vi "Drive Controller.vi"(8 "error in":errorcluster) -> ()   [LabVIEW 2020]
doc: "This VI executes continuously carrying out the current operation and responding to updates or new operation requests. It will often contain the timing or control code that is difficult to place directly in TeleOp. This VI generally opens all sensors and motors and isolates the rest of the robot code from knowing implementation details of how the operations are carried out."
uses:
  <vilib>/Rock Robotics/WPI/Framework/Completion Status.ctl
  Drive Setpoints.ctl
  Drive Operations.ctl
  Dawgma Programming Library/Controls/PurePursuit/RobotNeededPathData.ctl
  <vilib>/Rock Robotics/WPI/ThirdParty/REV Robotics/REVLib/Typedef/Spark MAX Sensor Type.ctl
  <vilib>/Rock Robotics/WPI/ThirdParty/REV Robotics/REVLib/Typedef/Spark MAX Idle Mode.ctl
  <vilib>/Rock Robotics/WPI/DriverStation/WPI_DriverStationRobotMode2.ctl
  <vilib>/Rock Robotics/WPI/ThirdParty/Sensors/navX/_TypeDefs/FRIC_navX_DeviceNumbersTypeDef.ctl
  <vilib>/Rock Robotics/WPI/ThirdParty/REV Robotics/REVLib/Typedef/Spark MAX Control Type.ctl
  Dawgma Programming Library/Controls/PurePursuit/PathFileData.ctl
  <vilib>/Rock Robotics/Network Tables/NT Write Variant.vi
  Configuration/Constants.vi
  <vilib>/Rock Robotics/Network Tables/NT Read Number.vi
  <vilib>/Rock Robotics/WPI/ThirdParty/Sensors/navX/_Processing Loop/FRIC_navX_Internal_SPI_ProcessingLoop.vi
panel:
  in  "Vel Convert":dbl=0.01786
  in  "Zero Encoders":bool
  out "Actual Angle":dbl=-174.33
  in  "Reset Loc & Ang":bool
  in  "Drive Conversion":dbl=1.75
  in  "SensorData":T1
  out "Graph":cluster{cluster{"x":dbl, "y":dbl}[]}[](graph)
  in  "PurePursuit Gains":T2={"FFV"=0.0097, "FFA"=0.002, "Vel PID"={"P"=0.0002, "I"=0.0, "D"=0.0}}
  out "Right Motor Out":dbl=0.1650746177556688
  out "Left Motor Out":dbl
  in  "SparkMAX PID":T3={"P"=0.038, "I"=0.0, "D"=0.0, "F"=0.001, "I Zone"=0.0, "Min Output"=-0.8, "Max Output"=0.8}
  in  "Interactive Values":T4={"Operation"=enum."Drive for Distance", "Left Setpoint"=0.1, "Right Setpoint"=0.1, "Duration"=100.0, "Distance"=300.0, "RobotNeededPathData"={"Path"=[], "MaxVel"=0.0, "MaxAccel"=0.0, "Backwards?"=FALSE, "PointSpacing"=0.0, "LookaheadDist"=0.0, "Speed/Curve"=1.8, "SlowDistanceAtEnd"=12.0, "SlowSpeed"=15.0, "MaxDeAccel"=0.0}, "PathFileName"="", "PathIndex"=0.0} {"RobotNeededPathData"."SlowSpeed" format="%#_13g"; "RobotNeededPathData"."SlowDistanceAtEnd" format="%#_13g"; "RobotNeededPathData"."Speed/Curve" format="%#_13g"}
  in  "Buttons":cluster{"Execute Cmd":bool, "Abort Cmd":bool}
  out "Command Timing":cluster{"Start Time (ms)":u32, "Iterations":i32}={"Start Time (ms)"=3589016, "Iterations"=0}
  out "Status":T7
  out "Current\nCmd":string="Started at  17:19:39.218\nDefault: Reserve,  L 0.0, R 0.0, D 0.000000"
  # "Tip: The graph shows the motor setpoints. It may also be helpful to observe inputs and sensor values.\nYou may also want to display tuning or debugging controls."
  # "THIS IS JUST\nFOR TESTING!"
  # "Interactive Command: You may fill in the settings for a command\nand schedule it with the Execute button. You can observe and abort\nany command while fine tuning the code for the controller."
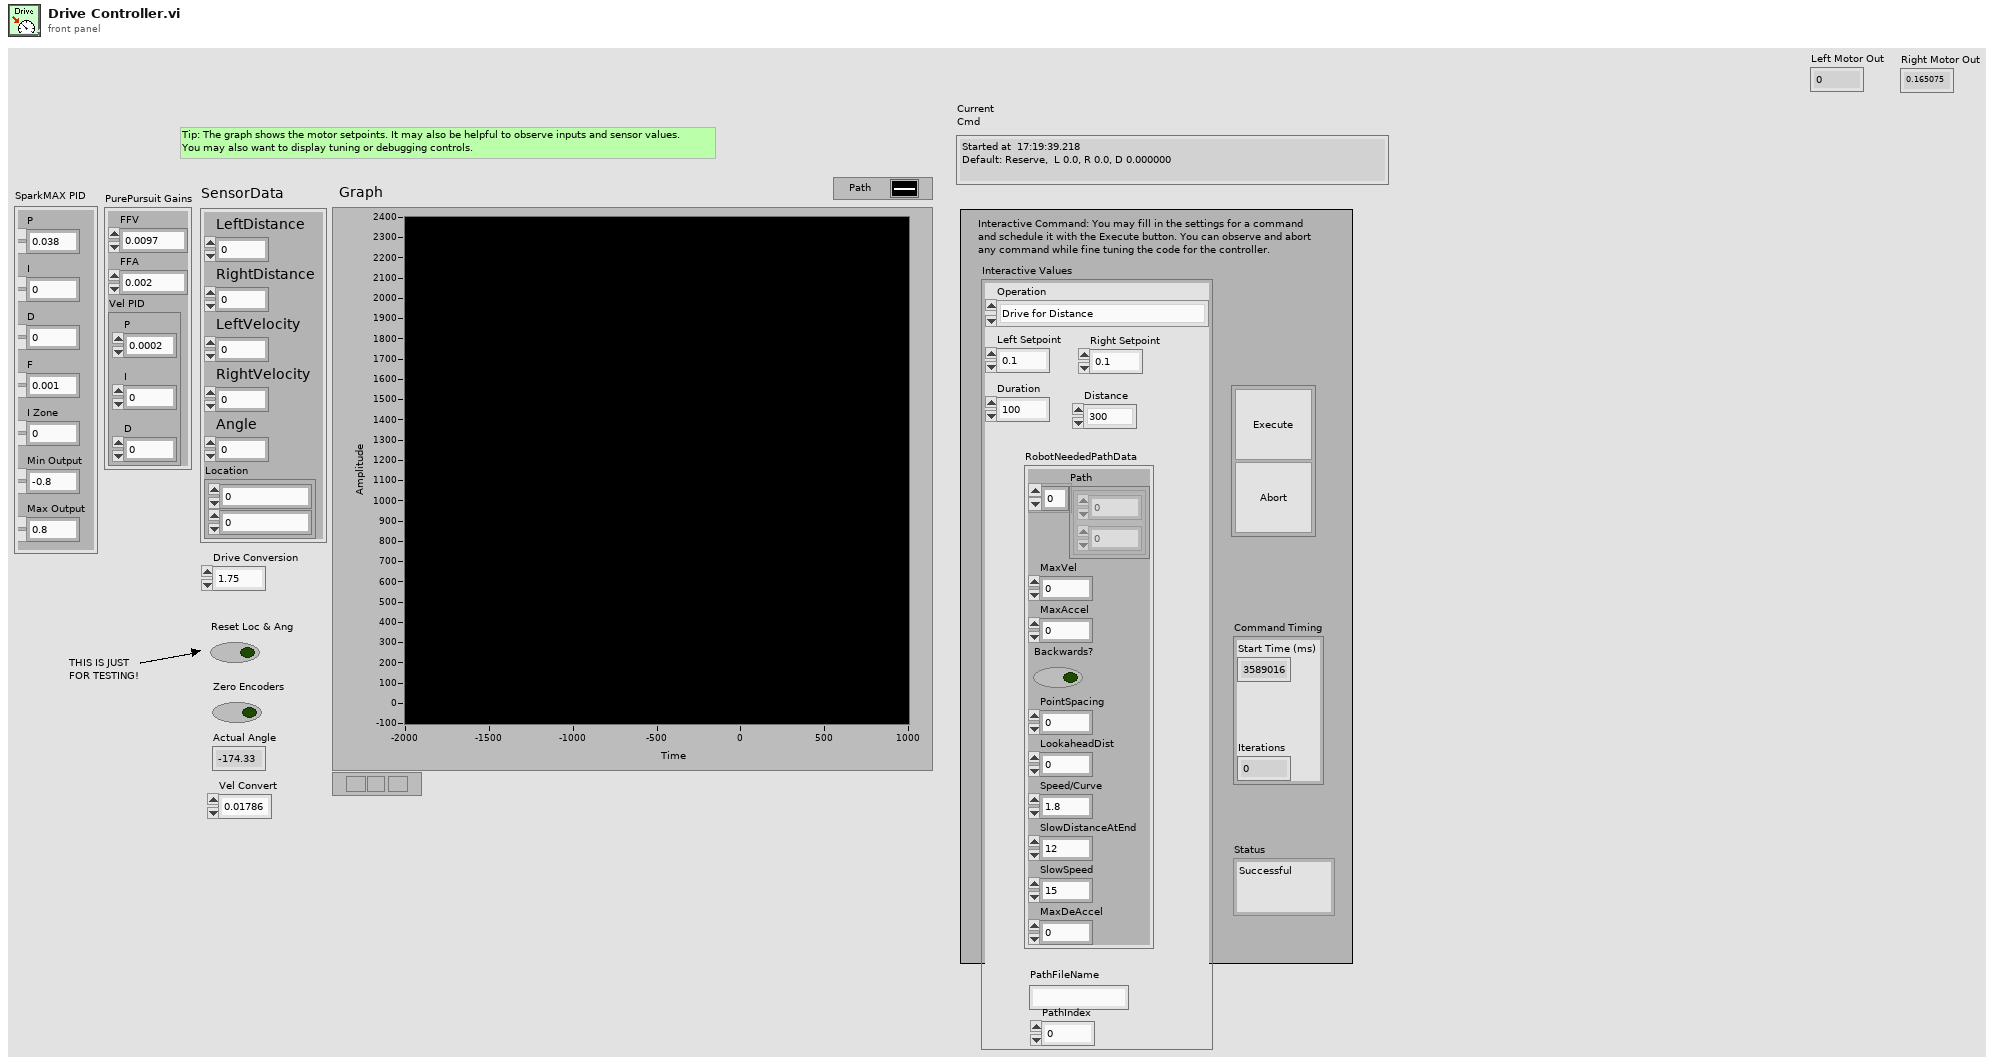
[diagram p1: front panel]
types:
  T1 = cluster{"LeftDistance":dbl, "RightDistance":dbl, "LeftVelocity":dbl, "RightVelocity":dbl, "Angle":dbl, "Location":cluster{dbl, dbl}}
  T2 = cluster{"FFV":dbl, "FFA":dbl, "Vel PID":cluster{"P":dbl, "I":dbl, "D":dbl}}
  T3 = cluster{"P":dbl, "I":dbl, "D":dbl, "F":dbl, "I Zone":dbl, "Min Output":dbl, "Max Output":dbl}
  T4 = typedef "Drive Setpoints.ctl" = cluster{"Operation":T5, "Left Setpoint":dbl, "Right Setpoint":dbl, "Duration":dbl, "Distance":dbl, "RobotNeededPathData":T6, "PathFileName":string, "PathIndex":dbl}
  T5 = typedef "Drive Operations.ctl" = enum16{"Reserve", "Read Current", "Immediate", "Drive for Time", "Drive for Distance", "AutoAlign", "Drive Path", "PurePursuitTest"}
  T6 = typedef "RobotNeededPathData.ctl" = cluster{"Path":cluster{dbl, dbl}[], "MaxVel":dbl, "MaxAccel":dbl, "Backwards?":bool, "PointSpacing":dbl, "LookaheadDist":dbl, "Speed/Curve":dbl, "SlowDistanceAtEnd":dbl, "SlowSpeed":dbl, "MaxDeAccel":dbl}
  T7 = typedef "Completion Status.ctl" = enum16{"Successful", "Aborted", "Incomplete"}
  T8 = typedef "Spark MAX Idle Mode.ctl" = enum16{"Coast", "Brake"}
  T9 = typedef "Spark MAX Sensor Type.ctl" = enum16{"No Sensor", "Hall Sensor", "Encoder", "-Not Available-", "Analog", "Alternate Encoder"}
  T10 = typedef "WPI_MotorControlDeviceRef.ctl" = cluster{"DeviceStatus":errorcluster, "Type":T11, "PWM":cluster{"PWM Channel":T12, "DeadBand":T13}, "CAN":cluster{"Device Number":u8, "SetOutput VI Ref":variant, "GetOutput VI Ref":variant, "Enable VI Ref":variant, "Disable VI Ref":variant, "Data":variant}, "Invert":bool, "DIO PWM":cluster{"PWM \"Enable\" Channel":T12, "DIOChannel":T14, "PWM Rate":dbl}}
  T11 = typedef "WPI_MotorControlType.ctl" = enum16{"PWM", "CAN", "DIO PWM"}
  T12 = typedef "FPGA_DIOPWMChannel.ctl" = enum8{"PWM 0", "PWM 1", "PWM 2", "PWM 3", "PWM 4", "PWM 5", "PWM 6", "PWM 7", "PWM 8", "PWM 9", "PWM MXP 0", "PWM MXP 1", "PWM MXP 2", "PWM MXP 3", "PWM MXP 4", "PWM MXP 5", "PWM MXP 6", "PWM MXP 7", "PWM MXP 8", "PWM MXP 9", "Invalid"}
  T13 = typedef "WPI_PWMDeadband.ctl" = cluster{"Name":string, "maxPositivePwm":i32, "minPositivePwm":i32, "centerPwm":i32, "maxNegativePwm":i32, "minNegativePwm":i32, "angularRange":u16}
  T14 = typedef "FPGA_DIOChannel.ctl" = enum8{"DIO 0", "DIO 1", "DIO 2", "DIO 3", "DIO 4", "DIO 5", "DIO 6", "DIO 7", "DIO 8", "DIO 9", "DIO MXP 0", "DIO MXP 1", "DIO MXP 2", "DIO MXP 3", "DIO MXP 4", "DIO MXP 5", "DIO MXP 6", "DIO MXP 7", "DIO MXP 8", "DIO MXP 9", "DIO MXP 10", "DIO MXP 11", "DIO MXP 12", "DIO MXP 13", "DIO MXP 14", "DIO MXP 15", "SPI Port CS1", "SPI Port CS2", "SPI Port CS3", "SPI Port MISO", "SPI Port MOSI", "Invalid"}
  T15 = typedef "Command Status Info.ctl" = cluster{"Name":string, "Status":T7, "notifier out":T16}
  T16 = typedef "Completion Notifier.ctl" = refnum<notifier>
  T17 = cluster{"SubSystem Data":T4, cluster{"Start Time (ms)":u32, "Iterations":i32}, cluster{"Command Info":T15, "Description":string, "Default Command":T4, "queue out":refnum<queue>, "Subsystem Name":string}}
  T18 = typedef "WPI_DriverStationRobotMode2.ctl" = enum16{"Autonomous Disabled", "Autonomous Enabled", "Teleop Disabled", "Teleop Enabled", "Disconnected", "Finish", "Test Disabled", "Test Enabled", "Emergency Stopped"}
  T19 = typedef "FRIC_navX_DeviceNumbersTypeDef.ctl" = enum16{"Dev0", "Dev1", "Dev2", "Dev3"}
  T20 = cluster{"Yaw":dbl, "Roll":dbl, "Pitch":dbl, "Heading":dbl, "Fused Heading":dbl}
  T21 = typedef "Spark MAX Control Type.ctl" = enum16{"Percent VBus", "Voltage", "Velocity", "Position", "Smart Motion", "Current", "Smart Velocity"}
  T22 = typedef "PathFileData.ctl" = cluster{"RobotNeeded":T6, "Meta":cluster{"Path (px)":cluster{i32, i32}[], "RobotWidth":dbl, "RobotLength":dbl, "CenterOfRotYOffset":dbl, "Roundedness":dbl, "StartingPositionPreset":u32, "PathName":string}}
  T23 = cluster{"SubSystem Data":T4, cluster{"Start Time (ms)":u32, "Iterations":i32}, "Default Command Arguments":cluster{"Command Info":T15, "Description":string, "Default Command":T4, "queue out":refnum<queue>, "Subsystem Name":string}}
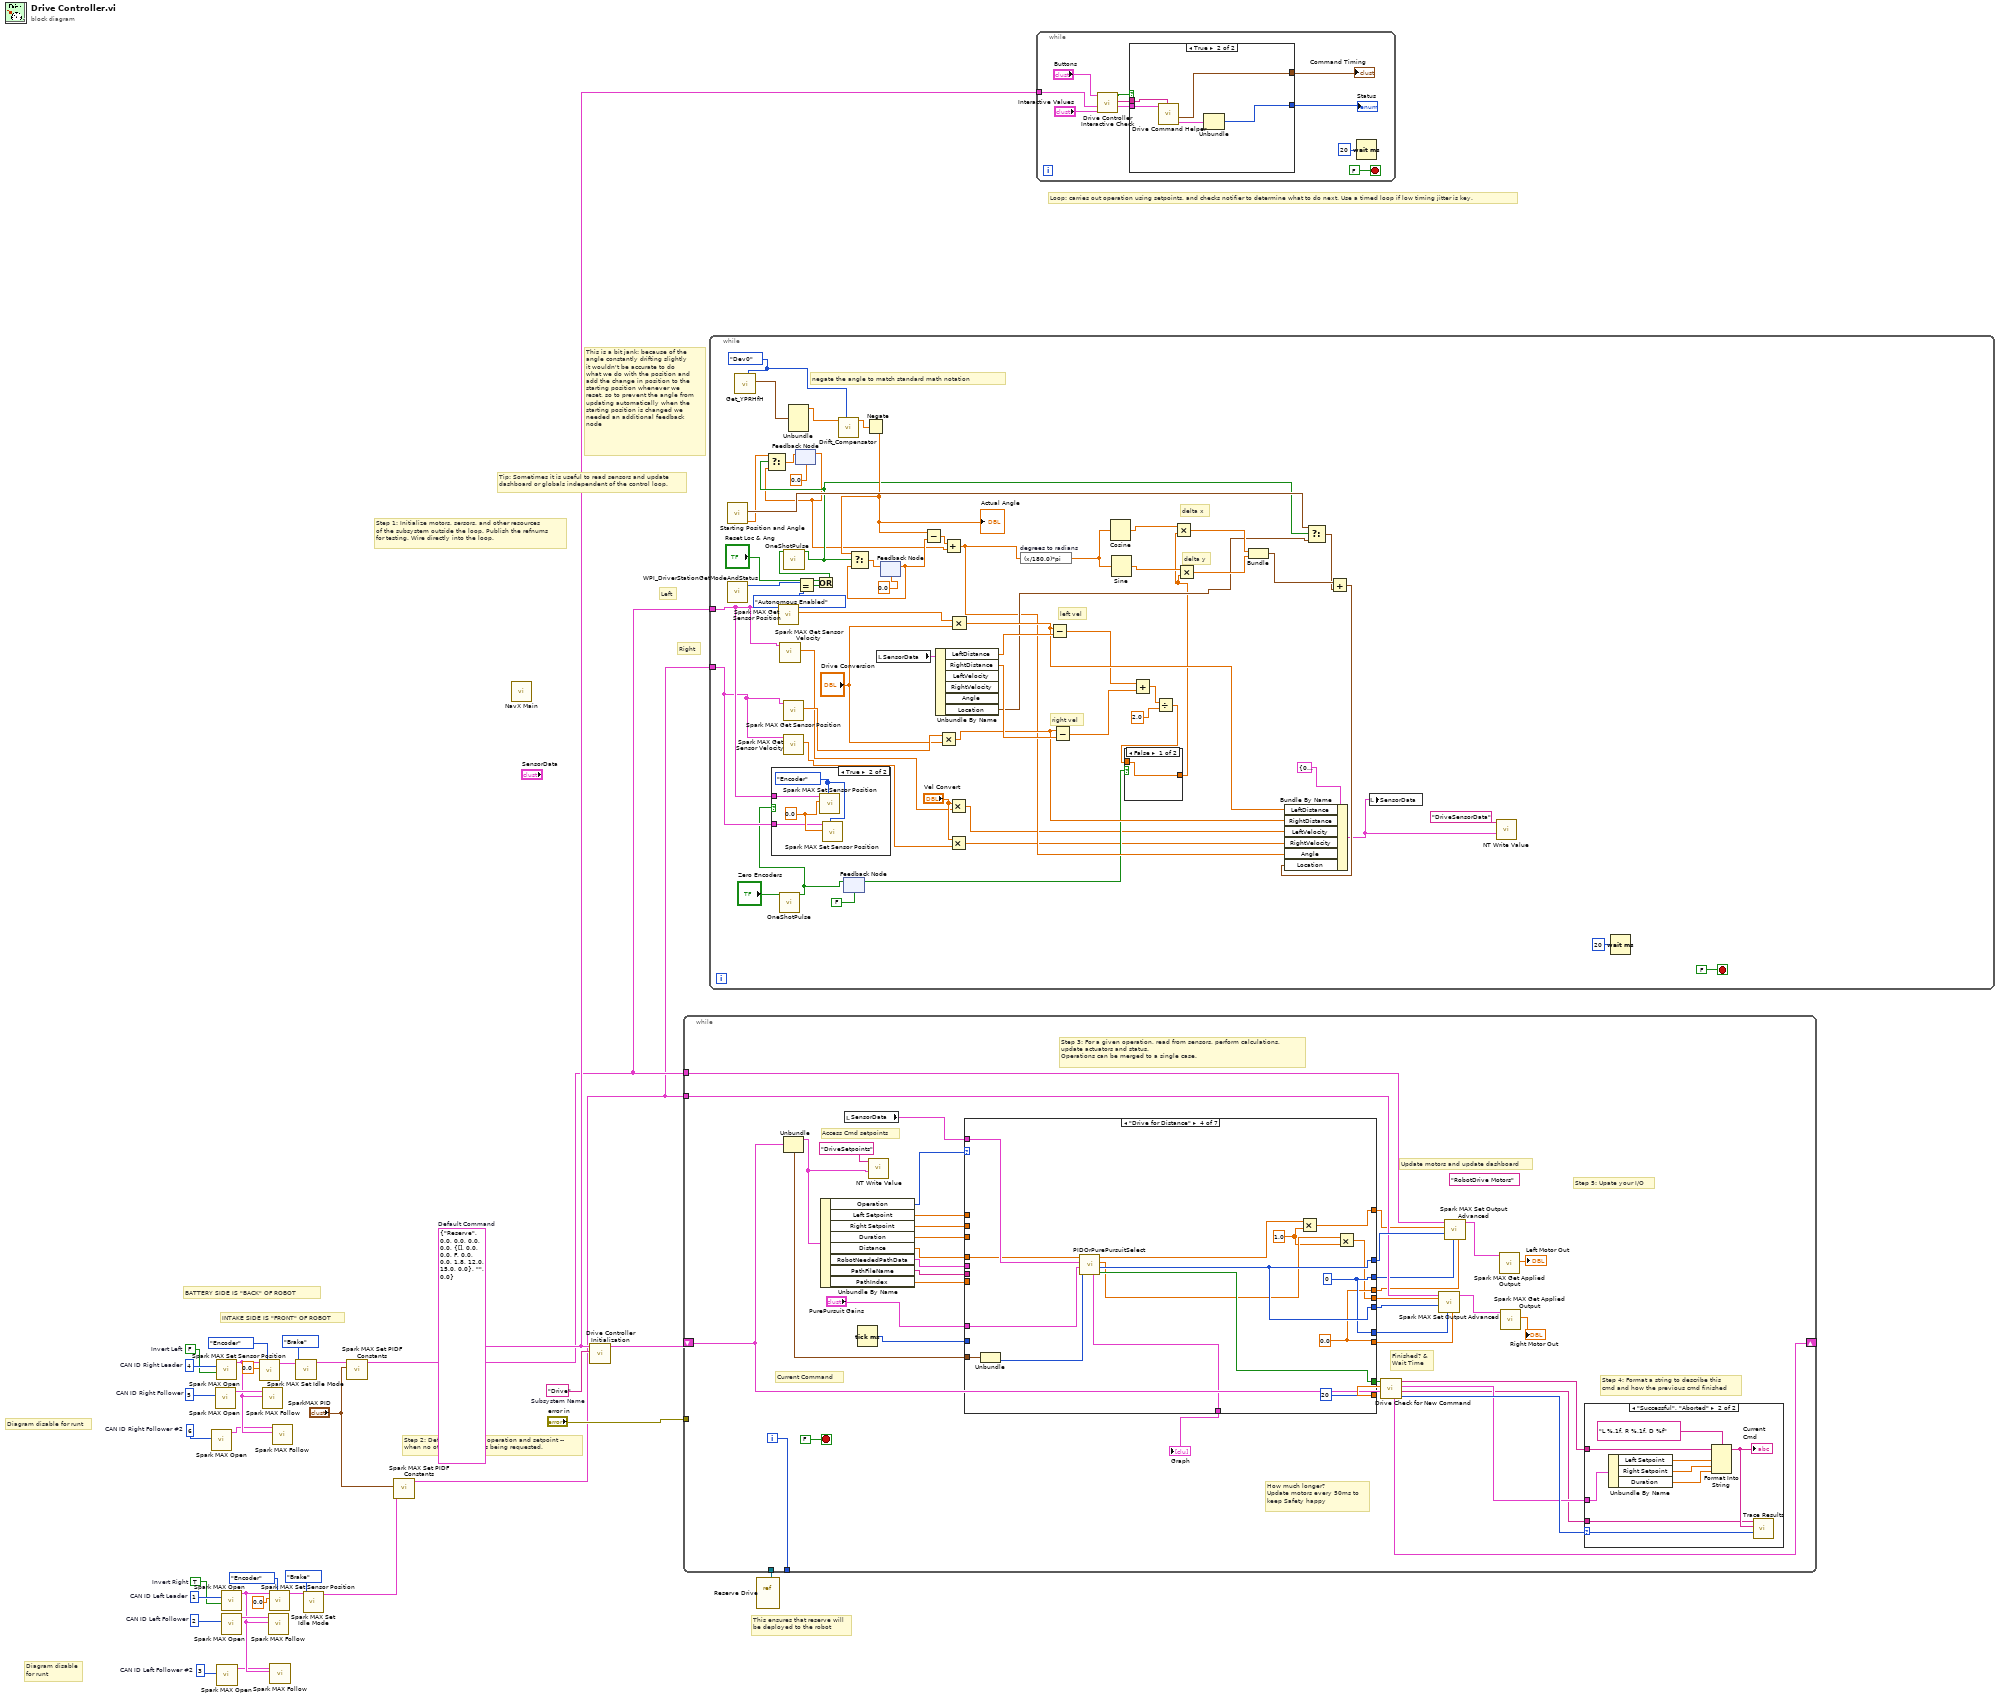
[diagram p0: block diagram]
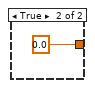
[diagram p2: hidden frame]
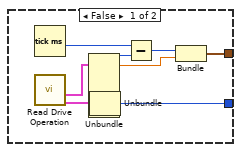
[diagram p4: hidden frame]
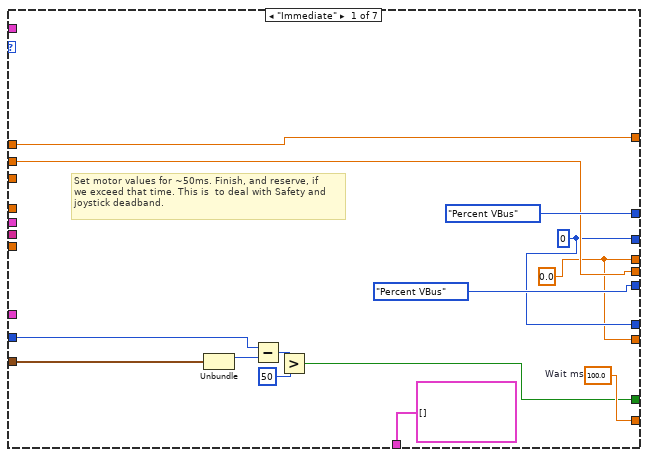
[diagram p6: hidden frame]
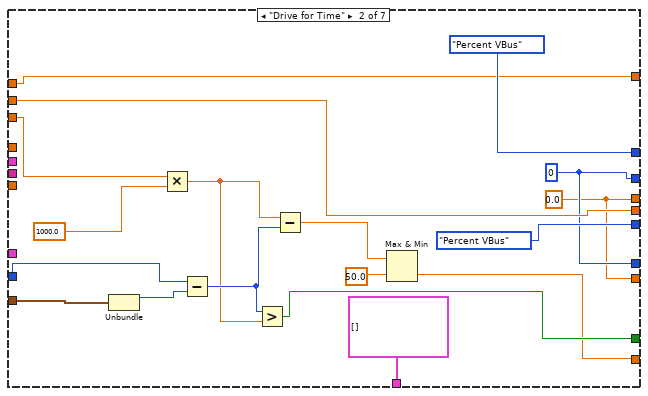
[diagram p7: hidden frame]
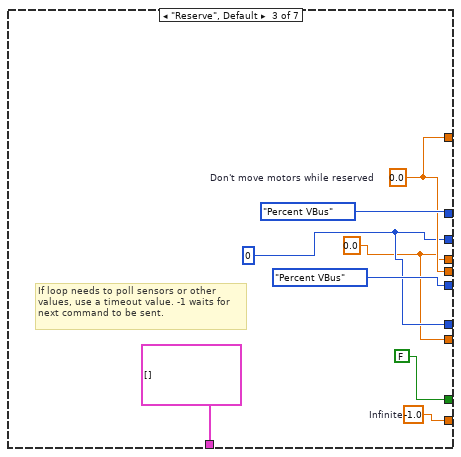
[diagram p8: hidden frame]
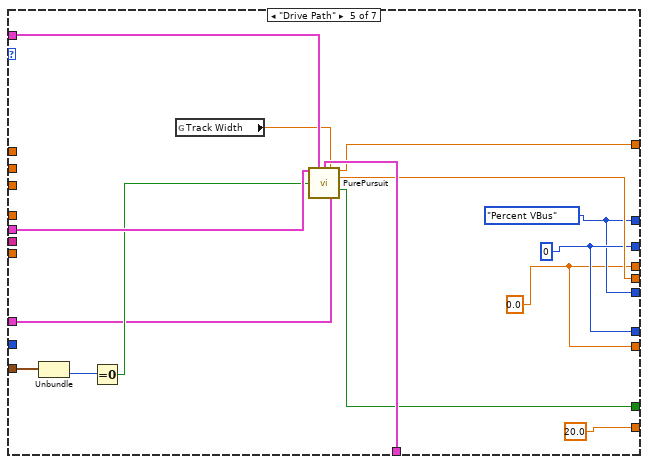
[diagram p9: hidden frame]
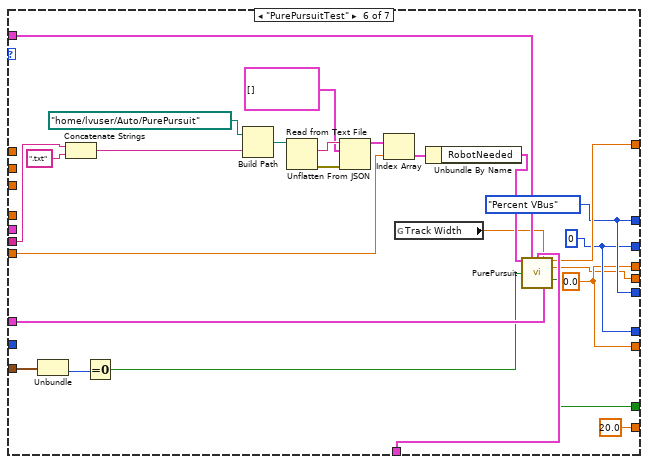
[diagram p10: hidden frame]
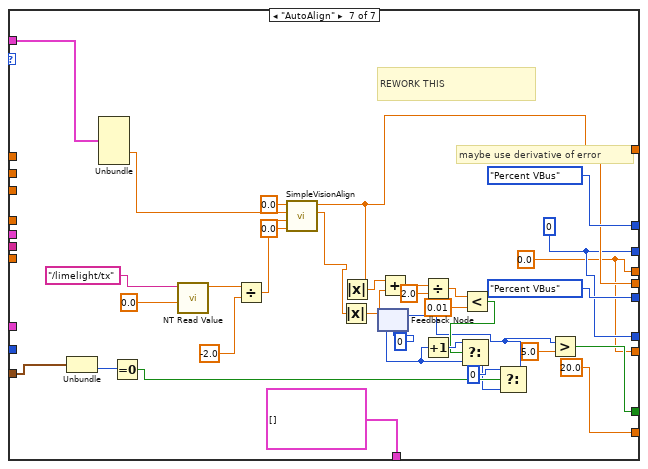
[diagram p11: hidden frame]
diagram:
  w2 = u8 3  # CAN ID Left Follower #2
  w4 = u8 6  # CAN ID Right Follower #2
  w9 = FALSE  # Invert Left
  w21 = TRUE  # Invert Right
  w23 = u8 1  # CAN ID Left Leader
  w22 = u8 2  # CAN ID Left Follower
  w26 = u8 4  # CAN ID Right Leader
  w27 = u8 5  # CAN ID Right Follower
  w28 = T4 {"Operation"=enum."Reserve", "Left Setpoint"=0.0, "Right Setpoint"=0.0, "Duration"=0.0, "Distance"=0.0, "RobotNeededPathData"={"Path"=[], "MaxVel"=0.0, "MaxAccel"=0.0, "Backwards?"=FALSE, "PointSpacing"=0.0, "LookaheadDist"=0.0, "Speed/Curve"=1.8, "SlowDistanceAtEnd"=12.0, "SlowSpeed"=15.0, "MaxDeAccel"=0.0}, "PathFileName"="", "PathIndex"=0.0}  # Default Command
  w32 = "Drive"  # Subsystem Name
  # "INTAKE SIDE IS \"FRONT\" OF ROBOT"
  # "This is a bit jank: because of the\nangle constantly drifting slightly\nit wouldn't be accurate to do\nwhat we do with the position and\nadd the change in position to the\nstarting position whenever we \nreset, so to prevent the angle from\nupdating automatically when the\nstarting position is changed we\nneeded an additional feedback\nnode"
  # "Diagram disable\nfor runt"
  # "Diagram disable for runt"
  # "BATTERY SIDE IS \"BACK\" OF ROBOT"
  # "Left"
  # "Right"
  # "This ensures that reserve will\nbe deployed to the robot"
  # "Tip: Sometimes it is useful to read sensors and update\ndashboard or globals independent of the control loop."
  # "Step 2: Define the default operation and setpoint --\nwhen no other operation is being requested."
  # "Step 1: Initialize motors, sersors, and other resources\nof the subsystem outside the loop. Publish the refnums\nfor testing. Wire directly into the loop."
  # "Loop: carries out operation using setpoints, and checks notifier to determine what to do next. Use a timed loop if low timing jitter is key."
  n1 = call <vilib>:"Spark MAX Open.vi"("Device Number"=w4) -> ("MotorControlDeviceRef"=w3:T10)  [unwired: 9 in, 1 out]
  n2 = call <vilib>:"Spark MAX Open.vi"("Device Number"=w27) -> ("MotorControlDeviceRef"=w25:T10)  [unwired: 9 in, 1 out]
  n3 = call <vilib>:"Spark MAX Open.vi"("Invert"=w9, "Device Number"=w26) -> ("MotorControlDeviceRef"=w7:T10)  [unwired: 8 in, 1 out]
  n4 = call <vilib>:"Spark MAX Open.vi"("Device Number"=w2) -> ("MotorControlDeviceRef"=w1:T10)  [unwired: 9 in, 1 out]
  n5 = call <vilib>:"Spark MAX Open.vi"("Invert"=w21, "Device Number"=w23) -> ("MotorControlDeviceRef"=w8:T10)  [unwired: 8 in, 1 out]
  n6 = call <vilib>:"Spark MAX Open.vi"("Device Number"=w22) -> ("MotorControlDeviceRef"=w24:T10)  [unwired: 9 in, 1 out]
  n7 = call <vilib>:"Spark MAX Set Sensor Position.vi"("Sensor Type (Hall Sensor)"=Spark_MAX_Sensor_Type."Encoder", "Position"=0.0, "MotorControlDeviceRef"=w7) -> ("MotorControlDeviceRef"=w17:T10)  [unwired: 7 in, 1 out]
  n8 = call <vilib>:"Spark MAX Follow.vi"("Master Controller"=w7, "MotorControlDeviceRef"=w25) -> ()  [unwired: 8 in, 2 out]
  n9 = call <vilib>:"Spark MAX Follow.vi"("Master Controller"=w8, "MotorControlDeviceRef"=w24) -> ()  [unwired: 8 in, 2 out]
  n10 = call <vilib>:"Spark MAX Set Sensor Position.vi"("Sensor Type (Hall Sensor)"=Spark_MAX_Sensor_Type."Encoder", "Position"=0.0, "MotorControlDeviceRef"=w8) -> ("MotorControlDeviceRef"=w16:T10)  [unwired: 7 in, 1 out]
  n11 = call <vilib>:"Spark MAX Follow.vi"("Master Controller"=w8, "MotorControlDeviceRef"=w1) -> ()  [unwired: 8 in, 2 out]
  n12 = call <vilib>:"Spark MAX Follow.vi"("Master Controller"=w7, "MotorControlDeviceRef"=w3) -> ()  [unwired: 8 in, 2 out]
  n13 = call <vilib>:"Spark MAX Set Idle Mode.vi"("Idle Mode"=Spark_MAX_Idle_Mode."Brake", "MotorControlDeviceRef in"=w17) -> ("MotorControlDeviceRef out"=w15:T10)  [unwired: 8 in, 1 out]
  n14 = call <vilib>:"Spark MAX Set Idle Mode.vi"("Idle Mode"=Spark_MAX_Idle_Mode."Brake", "MotorControlDeviceRef in"=w16) -> ("MotorControlDeviceRef out"=w14:T10)  [unwired: 8 in, 1 out]
  n15 = call <vilib>:"Spark MAX Set PIDF Constants.vi"("PID Constants"="SparkMAX PID", "MotorControlDeviceRef"=w15) -> ("MotorControlDeviceRef"=w11:T10)  [unwired: 8 in, 1 out]
  n16 = call <vilib>:"Spark MAX Set PIDF Constants.vi"("PID Constants"="SparkMAX PID", "MotorControlDeviceRef"=w14) -> ("MotorControlDeviceRef"=w10:T10)  [unwired: 8 in, 1 out]
  n17 = call-poly <vilib>:"NavX Main.vi"() -> ()  [unwired: 12 in]
  n18 = call "Drive Controller Initialization.vi"("Subsystem Name"=w32, "Default Command"=w28) -> ("Current Command"=w30:T17)  [unwired: 9 in]
  n19 = while {
    tunnel: w11 -> [w55]
    tunnel: w10 -> [w54]
    stop <- FALSE stop-if-true
    w38 = FRIC_navX_DeviceNumbersTypeDef."Dev0" ("Device Number")
    # "negate the angle to match standard math notation"
    # "delta y"
    # "delta x"
    # "right vel"
    # "left vel"
    n20 = call "Starting Position and Angle.vi"() -> ("Angle"=w35:dbl, "Location"=w61:cluster{"X":dbl, "Y":dbl})  [unwired: 10 in]
    n21 = call <vilib>:"WPI_DriverStationGetModeAndStatus.vi"() -> ("Robot Mode"=w65:T18)  [unwired: 10 in, 1 out]
    n22 = call <vilib>:"Get_YPRHfH.vi"("Device Number"=w38) -> ("YRPHfH"=w90:T20)  [unwired: 10 in]
    n23 = call <vilib>:"Spark MAX Get Sensor Position.vi"("MotorControlDevRef in"=w55) -> ("Sensor Position"=w77:dbl)  [unwired: 7 in, 3 out]
    n24 = call "OneShotPulse.vi"("Input"="Zero Encoders") -> ("Output"=w52:bool)  [unwired: 10 in]
    n25 = case shown="True" w52 {
      tunnel: w55 -> [_ w97]
      tunnel: w54 -> [_ w96]
      frame False {
      }
      frame True {
        w95 = Spark_MAX_Sensor_Type."Encoder" ("Sensor Type (Hall Sensor)")
        w98 = 0.0
        n26 = call <vilib>:"Spark MAX Set Sensor Position.vi"("Sensor Type (Hall Sensor)"=w95, "Position"=w98, "MotorControlDeviceRef"=w97) -> ()  [unwired: 7 in, 2 out]
        n27 = call <vilib>:"Spark MAX Set Sensor Position.vi"("Sensor Type (Hall Sensor)"=w95, "Position"=w98, "MotorControlDeviceRef"=w96) -> ()  [unwired: 7 in, 2 out]
      }
    }
    n28 = call <vilib>:"Spark MAX Get Sensor Velocity.vi"("MotorControlDevRef in"=w55) -> ("Sensor Velocity"=w44:dbl)  [unwired: 7 in, 3 out]
    n29 = call <vilib>:"Spark MAX Get Sensor Position.vi"("MotorControlDevRef in"=w54) -> ("Sensor Position"=w75:dbl)  [unwired: 7 in, 3 out]
    n30 = call <vilib>:"Spark MAX Get Sensor Velocity.vi"("MotorControlDevRef in"=w54) -> ("Sensor Velocity"=w43:dbl)  [unwired: 7 in, 3 out]
    n31 = Unbundle(w90) -> ("Yaw"=w40:dbl)  [unwired: 4 out]
    n32 = feedback #1(0.0) -> (w33:dbl)
    n33 = Equal?(x=w65, y=WPI_DriverStationRobotMode2."Autonomous Enabled" ("Robot Mode")) -> (x = y?=w67:bool)
    n34 = Or(x="Reset Loc & Ang", y=w67) -> (x .or. y?=w68:bool)
    n35 = call "OneShotPulse.vi"("Input"=w68) -> ("Output"=w36:bool)  [unwired: 10 in]
    n36 = Select(t=w35, s=w36, f=w33) -> (s? t:f=w34:dbl)
    n37 = feedback-in #1(w34) -> ()
    n38 = call <vilib>:"Drift_Compensator.vi"("Device Number"=w38, "Raw Yaw"=w40) -> ("comp yaw"=w39:dbl)  [unwired: 9 in]
    n39 = feedback-in #2(w52) -> ()
    n40 = feedback #2(FALSE ("Output")) -> (w50:bool)
    n41 = Negate(x=w39) -> (-x=w57:dbl)
    "Actual Angle" <- w57
    n42 = local read "SensorData"() -> (w89:T1)
    n43 = feedback #3(0.0) -> (w59:dbl)
    n44 = Select(t=w57, s=w36, f=w59) -> (s? t:f=w58:dbl)
    n45 = feedback-in #3(w58) -> ()
    n46 = Subtract(x=w57, y=w59) -> (x-y=w60:dbl)
    n47 = Unbundle By Name(w89) -> ("LeftDistance"=w88:dbl, "RightDistance"=w87:dbl, "Location"=w63:cluster{dbl, dbl})  [unwired: 3 out]
    n48 = Multiply(x=w75, y="Drive Conversion") -> (x*y=w73:dbl)
    n49 = Add(x=w60, y=w33) -> (x+y=w56:dbl)
    n50 = Multiply(x="Vel Convert", y=w44) -> (x*y=w42:dbl)
    n51 = Multiply(x="Vel Convert", y=w43) -> (x*y=w41:dbl)
    n52 = Multiply(x=w77, y="Drive Conversion") -> (x*y=w76:dbl)
    n53 = expression code="(x/180.0)*pi" "degrees to radians"(w56) -> (w70:dbl)
    n54 = Subtract(x=w76, y=w88) -> (x-y=w47:dbl)
    n55 = Subtract(x=w73, y=w87) -> (x-y=w46:dbl)
    n56 = Cosine(x=w70) -> (cos(x)=w82:dbl)
    n57 = Sine(x=w70) -> (sin(x)=w83:dbl)
    n58 = Add(x=w47, y=w46) -> (x+y=w84:dbl)
    n59 = Divide(x=w84, y=2.0) -> (x/y=w49:dbl)
    n60 = case shown="False" w50 {
      tunnel: [w93 0.0] -> w48
      tunnel: w49 -> [w93 _]
      frame False {
      }
      frame True {
      }
    }
    n61 = Multiply(x=w82, y=w48) -> (x*y=w80:dbl)
    n62 = Multiply(x=w83, y=w48) -> (x*y=w81:dbl)
    n63 = Bundle(w80, w81) -> (w79:cluster{dbl, dbl})  [unwired: 1 in]
    n64 = Select(t=w61, s=w36, f=w63) -> (s? t:f=w62:cluster{"X":dbl, "Y":dbl})
    n65 = Add(x=w79, y=w62) -> (x+y=w78:cluster{dbl, dbl})
    n66 = Bundle By Name(cluster=T1 {"LeftDistance"=0.0, "RightDistance"=0.0, "LeftVelocity"=0.0, "RightVelocity"=0.0, "Angle"=0.0, "Location"={0.0, 0.0}} ("SensorData"), "LeftDistance"=w76, "RightDistance"=w73, "LeftVelocity"=w42, "RightVelocity"=w41, "Angle"=w56, "Location"=w78) -> (w71:T1)
    n67 = local write "SensorData"(w71) -> ()
    n68 = call-poly <vilib>:"NT Write Value.vi"("Variant"=w71, "Name"="DriveSensorData") -> ()  [unwired: 9 in, 1 out]
    n69 = Wait (ms)(milliseconds to wait=20) -> ()  [unwired: 1 out]
  }
  n70 = vi-ref "Reserve Drive.vi"() -> (w29:refnum<vi>)
  n71 = while {
    shift-right: [w133] -> _
    shift-left: w30 -> [w127]
    tunnel: [w136] -> _
    tunnel: "error in" -> [_]
    tunnel: w29 -> [_]
    tunnel: w11 -> [w118]
    tunnel: w10 -> [w117]
    i -> [w136]
    stop <- FALSE stop-if-true
    (unwired) "RobotDrive Motors" ("Name")
    # "How much longer?\nUpdate motors every 50ms to\nkeep Safety happy"
    # "Step 5: Upate your I/O"
    # "Step 4: Format a string to describe this\ncmd and how the previous cmd finished"
    # "Current Command"
    # "Update motors and update dashboard"
    # "Access Cmd setpoints"
    # "Finished? &\nWait Time"
    # "Step 3: For a given operation, read from sensors, perform calculations,\nupdate actuators and status.\nOperations can be merged to a single case."
    n72 = Unbundle(w127) -> ("SubSystem Data"=w105:T4, w128:cluster{"Start Time (ms)":u32, "Iterations":i32})  [unwired: 1 out]
    n73 = Unbundle By Name(w105) -> ("Operation"=w111:T5, "Left Setpoint"=w110:dbl, "Right Setpoint"=w109:dbl, "Duration"=w107:dbl, "Distance"=w108:dbl, "RobotNeededPathData"=w106:T6, "PathFileName"=w102:string, "PathIndex"=w101:dbl)
    n74 = local read "SensorData"() -> (w112:T1)
    n75 = Tick Count (ms)() -> (millisecond timer value=w135:u32)
    n76 = call-poly <vilib>:"NT Write Value.vi"("Variant"=w105, "Name"="DriveSetpoints") -> ()  [unwired: 9 in, 1 out]
    n77 = case shown="\"Drive for Distance\"" w111 {
      tunnel: [w160 w161 w186 20 ("PIDF Slot (0)") 20.0 20.0 ("Infinite") 20.0 ("Infinite")] -> w132
      tunnel: w128 -> [w155 w178 _ w195 w216 w224 w253]
      tunnel: w135 -> [w156 w176 _ _ _ _ _]
      tunnel: "PurePursuit Gains" -> [_ _ _ w202 w211 w225 _]
      tunnel: [cluster{cluster{"x":dbl, "y":dbl}[]}[] [] ("Graph") cluster{cluster{"x":dbl, "y":dbl}[]}[] [] ("Graph") cluster{cluster{"x":dbl, "y":dbl}[]}[] [] ("Graph") w200 w213 w230 cluster{cluster{"x":dbl, "y":dbl}[]}[] [] ("Graph")] -> w121
      tunnel: [w148 w163 w180 w193 w206 w220 w245] -> w116
      tunnel: [w147 w162 w179 w192 w204 w219 w244] -> w114
      tunnel: [w148 w163 w180 w193 w206 w220 w245] -> w113
      tunnel: [w147 w162 w179 w192 w204 w219 w244] -> w120
      tunnel: [Spark_MAX_Control_Type."Percent VBus" ("Control Mode") Spark_MAX_Control_Type."Percent VBus" ("Control Mode") Spark_MAX_Control_Type."Percent VBus" ("Control Mode") w197 w205 w221 Spark_MAX_Control_Type."Percent VBus" ("Control Mode")] -> w119
      tunnel: [w150 w166 w181 w190 w209 w228 w246] -> w100
      tunnel: [Spark_MAX_Control_Type."Percent VBus" ("Control Mode") Spark_MAX_Control_Type."Percent VBus" ("Control Mode") Spark_MAX_Control_Type."Percent VBus" ("Control Mode") w197 w205 w221 Spark_MAX_Control_Type."Percent VBus" ("Control Mode")] -> w115
      tunnel: [w149 w165 w181 w188 w208 w218 w246] -> w99
      tunnel: [w151 w168 FALSE ("ignore previous (F)") w198 w212 w227 w250] -> w103
      tunnel: w112 -> [_ _ _ w201 w210 w231 w254]
      tunnel: w110 -> [w150 w166 _ _ _ _ _]
      tunnel: w109 -> [w149 w165 _ _ _ _ _]
      tunnel: w108 -> [_ _ _ w196 _ _ _]
      tunnel: w107 -> [_ w164 _ _ _ _ _]
      tunnel: w106 -> [_ _ _ _ w217 _ _]
      tunnel: w102 -> [_ _ _ _ _ w234 _]
      tunnel: w101 -> [_ _ _ _ _ w233 _]
      frame "Immediate" {
        w147 = 0.0
        w148 = 0
        w160 = 100.0  # Wait ms
        # "Set motor values for ~50ms. Finish, and reserve, if\nwe exceed that time. This is  to deal with Safety and\njoystick deadband."
        n78 = Unbundle(w155) -> ("Start Time (ms)"=w157:u32)  [unwired: 1 out]
        n79 = Subtract(x=w156, y=w157) -> (x-y=w158:u32)
        n80 = Greater?(x=w158, y=u8 50 ("Left Motor")) -> (0:w151:bool)
      }
      frame "Drive for Time" {
        w162 = 0.0
        w163 = 0
        n81 = Unbundle(w178) -> ("Start Time (ms)"=w177:u32)  [unwired: 1 out]
        n82 = Multiply(x=w164, y=1000.0) -> (x*y=w169:dbl)
        n83 = Subtract(x=w176, y=w177) -> (x-y=w170:u32)
        n84 = Greater?(x=w170, y=w169) -> (0:w168:bool)
        n85 = Subtract(x=w169, y=w170) -> (x-y=w167:dbl)
        n86 = Max & Min(x=w167, y=50.0) -> (min(x,y)=w161:dbl)  [unwired: 1 out]
      }
      frame "Reserve", Default {
        w179 = 0.0
        w180 = 0
        w181 = 0.0  # Don't move motors while reserved
        w186 = -1.0  # Infinite
        # "If loop needs to poll sensors or other\nvalues, use a timeout value. -1 waits for\nnext command to be sent."
      }
      frame "Drive for Distance" {
        w187 = 1.0
        w192 = 0.0
        w193 = 0 ("PIDF Slot (0)")
        n87 = Unbundle(w195) -> ("Iterations"=w194:i32)  [unwired: 1 out]
        n88 = call "PIDOrPurePursuitSelect.vi"("Distance"=w196, "SensorData"=w201, "PurePursuit Gains"=w202, "Iterations"=w194) -> ("Graph"=w200:cluster{cluster{"x":dbl, "y":dbl}[]}[], "Left Output"=w191:dbl, "Right Output"=w189:dbl, "Control Mode"=w197:T21, "Done?"=w198:bool)  [unwired: 2 in]
        n89 = Multiply(x=w191, y=w187) -> (x*y=w190:dbl)
        n90 = Multiply(x=w189, y=w187) -> (x*y=w188:dbl)
      }
      frame "Drive Path" {
        w204 = 0.0
        w206 = 0
        w205 = Spark_MAX_Control_Type."Percent VBus" ("Control Mode")
        n91 = Unbundle(w216) -> ("Iterations"=w215:i32)  [unwired: 1 out]
        n92 = Equal To 0?(x=w215) -> (x = 0?=w214:bool)
        n93 = global read "Constants.vi" "Track Width"() -> (w203:dbl)
        n94 = call "PurePursuit.vi"("RobotNeededPathData"=w217, "SensorData"=w210, "Trackwidth"=w203, "Reset"=w214, "Gains"=w211) -> ("Graph"=w213:cluster{cluster{"x":dbl, "y":dbl}[]}[], "LeftValue"=w209:dbl, "RightValue"=w208:dbl, "Done"=w212:bool)  [unwired: 6 in, 1 out]
      }
      frame "PurePursuitTest" {
        w219 = 0.0
        w220 = 0
        w221 = Spark_MAX_Control_Type."Percent VBus" ("Control Mode")
        n95 = Unbundle(w224) -> ("Iterations"=w223:i32)  [unwired: 1 out]
        n96 = Concatenate Strings(w234, ".txt" ("string")) -> (w242:string)
        n97 = Equal To 0?(x=w223) -> (x = 0?=w222:bool)
        n98 = Build Path(base path=path "/home/lvuser/Auto/PurePursuit", name or relative path=w242) -> (appended path=w240:path)
        n99 = Read from Text File(file (use dialog)=w240) -> (text=w238:string, error out=w239:errorcluster)  [unwired: 3 in, 2 out]
        n100 = Unflatten From JSON(JSON string=w238, type and defaults=T22[] [], error in (no error)=w239) -> (value=w236:T22[])  [unwired: 4 in, 1 out]
        n101 = Index Array(array=w236, index=w233) -> (element=w235:T22)
        n102 = global read "Constants.vi" "Track Width"() -> (w229:dbl)
        n103 = Unbundle By Name(w235) -> ("RobotNeeded"=w232:T6)
        n104 = call "PurePursuit.vi"("RobotNeededPathData"=w232, "SensorData"=w231, "Trackwidth"=w229, "Reset"=w222, "Gains"=w225) -> ("Graph"=w230:cluster{cluster{"x":dbl, "y":dbl}[]}[], "LeftValue"=w228:dbl, "RightValue"=w218:dbl, "Done"=w227:bool)  [unwired: 6 in, 1 out]
      }
      frame "AutoAlign" {
        w244 = 0.0
        w245 = 0 ("PIDF Slot (0)")
        # "maybe use derivative of error"
        # "REWORK THIS"
        n105 = Unbundle(w253) -> ("Iterations"=w259:i32)  [unwired: 1 out]
        n106 = Unbundle(w254) -> ("Angle"=w278:dbl)  [unwired: 5 out]
        n107 = Equal To 0?(x=w259) -> (x = 0?=w258:bool)
        n108 = call-poly <vilib>:"NT Read Value.vi"("Default Value"=0.0, "Name"="/limelight/tx") -> ("Numeric"=w275:dbl)  [unwired: 8 in, 1 out]
        n109 = Divide(x=w275, y=-2.0) -> (x/y=w273:dbl)
        n110 = call "SimpleVisionAlign.vi"("Manual Turn"=0.0, "Target Offset"=w273, "Gyro Angle"=w278, "Throttle"=0.0) -> ("Right Power"=w247:dbl, "Left Power"=w246:dbl)  [unwired: 6 in]
        n111 = Absolute Value(x=w247) -> (abs(x)=w268:dbl)
        n112 = Absolute Value(x=w246) -> (abs(x)=w267:dbl)
        n113 = feedback #4(0) -> (w261:i32)
        n114 = Add(x=w267, y=w268) -> (x+y=w266:dbl)
        n115 = Divide(x=w266, y=2.0) -> (x/y=w264:dbl)
        n116 = Increment(x=w261) -> (x+1=w262:i32)
        n117 = Less?(x=w264, y=0.01) -> (x < y?=w260:bool)
        n118 = Select(t=w262, s=w260, f=w261) -> (s? t:f=w256:i32)
        n119 = Select(t=0, s=w258, f=w256) -> (s? t:f=w255:i32)
        n120 = feedback-in #4(w255) -> ()
        n121 = Greater?(x=w255, y=5.0) -> (0:w250:bool)
      }
    }
    "Graph" <- w121
    n122 = call "Drive Check for New Command.vi"("input cluster"=w127, "Wait time (ms)"=w132, "Finished?"=w103) -> ("Completion"=w134:T7, "Subsystem Name"=w129:string, "Current Command"=w130:T4, "Initial Trace String"=w131:string, "Next Command"=w133:T23)  [unwired: 4 in]
    n123 = call <vilib>:"Spark MAX Set Output Advanced.vi"("Arbitrary Feed Forward (0)"=w120, "PIDF Slot (0)"=w116, "Control Mode"=w115, "Setpoint"=w99, "MotorControlDevRef"=w117) -> ("MotorControlDevRef"=w124:T10)  [unwired: 5 in, 1 out]
    n124 = call <vilib>:"Spark MAX Set Output Advanced.vi"("Arbitrary Feed Forward (0)"=w114, "PIDF Slot (0)"=w113, "Control Mode"=w119, "Setpoint"=w100, "MotorControlDevRef"=w118) -> ("MotorControlDevRef"=w126:T10)  [unwired: 5 in, 1 out]
    n125 = call <vilib>:"Spark MAX Get Applied Output.vi"("MotorControlDevRef in"=w126) -> ("Applied Output"=→"Left Motor Out":dbl)  [unwired: 7 in, 3 out]
    n126 = call <vilib>:"Spark MAX Get Applied Output.vi"("MotorControlDevRef in"=w124) -> ("Applied Output"=→"Right Motor Out":dbl)  [unwired: 7 in, 3 out]
    n127 = case shown="\"Successful\", \"Aborted\"" w134 {
      selector: w134 -> [_ w146]
      tunnel: w131 -> [_ w141]
      tunnel: w130 -> [_ w142]
      tunnel: w129 -> [_ w138]
      frame "Incomplete", Default {
        # "Continuing current command"
      }
      frame "Successful", "Aborted" {
        # "Report and setup for next command"
        n128 = Unbundle By Name(w142) -> ("Left Setpoint"=w144:dbl, "Right Setpoint"=w145:dbl, "Duration"=w139:dbl)
        n129 = Format Into String(format string="L %.1f, R %.1f, D %f", initial string=w141, w144, w145, w139) -> (resulting string=w140:string)  [unwired: 1 in, 1 out]
        "Current\nCmd" <- w140
        n130 = call <vilib>:"Trace Results.vi"("Status of previous command"=w146, "Description"=w140, "Subsystem"=w138) -> ()  [unwired: 9 in]
      }
    }
  }
  n131 = while {
    tunnel: w28 -> [w280]
    stop <- FALSE stop-if-true
    n132 = call "Drive Controller Interactive Check.vi"("Interactive Command In"="Interactive Values", "Default Command"=w280, "Buttons"="Buttons") -> ("Interactive Command Out"=w282:T4, "Trace String"=w283:string, "Schedule"=w284:bool)  [unwired: 6 in]
    n133 = case shown="True" w284 {
      tunnel: [w293 w301] -> w285
      tunnel: [w292 w297] -> w286
      tunnel: w283 -> [_ w299]
      tunnel: w282 -> [_ w298]
      frame False {
        n134 = Tick Count (ms)() -> (millisecond timer value=w296:u32)
        n135 = call "Read Drive Operation.vi"() -> ("Command Info"=w290:T15, "SubSystem Data"=w289:T4)  [unwired: 9 in, 1 out]
        n136 = Unbundle(w289) -> ("Operation"=w294:T5, "Left Setpoint"=w291:dbl)  [unwired: 6 out]
        n137 = Unbundle(w290) -> ("Status"=w293:T7)  [unwired: 2 out]
        n138 = Subtract(x=w296, y=w294) -> (x-y=w295:u32)
        n139 = Bundle(w295, "Left Setpoint"=w291) -> (w292:cluster{u32, "Left Setpoint":dbl})  [unwired: 1 in]
      }
      frame True {
        n140 = call "Drive Command Helper.vi"("Description"=w299, "SubSystem Data"=w298) -> ("Command Info Out"=w300:T15, "Command Timing"=w297:cluster{"Start Time (ms)":u32, "Iterations":i32})  [unwired: 7 in, 1 out]
        n141 = Unbundle(w300) -> ("Status"=w301:T7)  [unwired: 2 out]
      }
    }
    "Status" <- w285
    "Command Timing" <- w286
    n142 = Wait (ms)(milliseconds to wait=u32 20) -> ()  [unwired: 1 out]
  }
